vi "Function.vi"(8 "error in (no error)":errorcluster, 9 "Bool B":bool[](array[boolean]), 10 "Bool A":bool[](array[boolean]), 11 "Two Terminal in":refnum<class "AbsFunc_Two Term_Bool_1D.lvclass">) -> (0 "error out":errorcluster, 2 "Result":bool[](array[boolean]), 3 "Two Terminal out":refnum<class "AbsFunc_Two Term_Bool_1D.lvclass">)   [LabVIEW 2021, in "AbsFunc_Two Term_Bool_1D.lvclass"]
uses:
  AbsFunc_Two Term_Bool_1D.lvclass
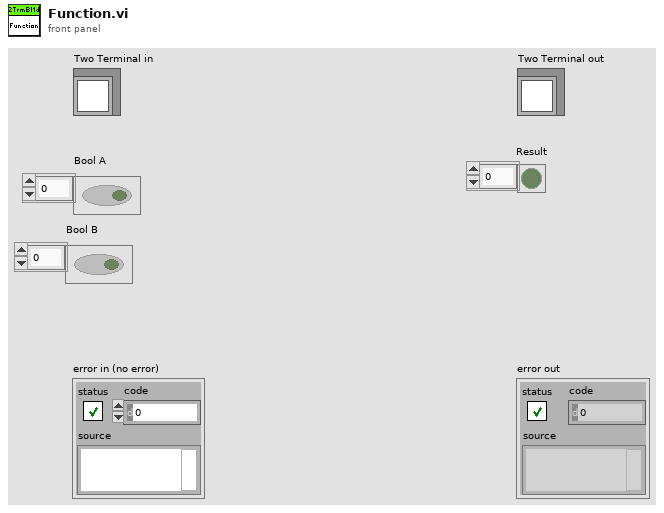
[diagram p1: front panel]
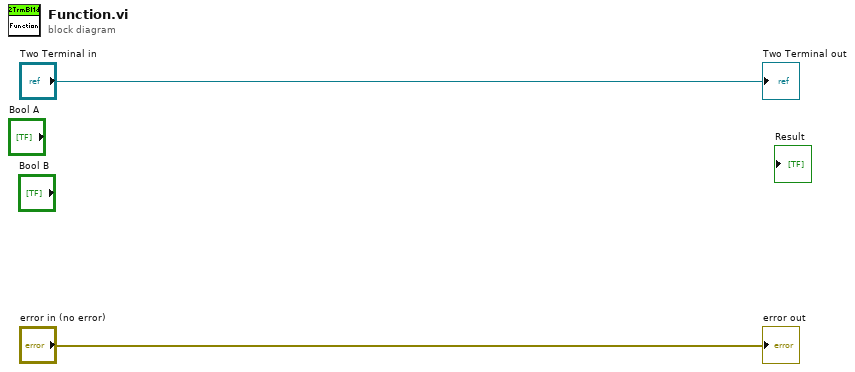
[diagram p0: block diagram]
diagram:
  "error out" <- "error in (no error)"
  "Two Terminal out" <- "Two Terminal in"
